vi "Global 2.vi"() -> ()   [LabVIEW 2015]
panel:
  in  "Stop Button":bool
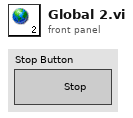
[diagram p1: front panel]
diagram:
